vi "Dispose.vi"(8 "error in (no error)":errorcluster, 11 "STOMP in":refnum<class "STOMP.lvclass">) -> (0 "error out":errorcluster, 3 "STOMP out":refnum<class "STOMP.lvclass">)   [LabVIEW 2017, in "STOMP.lvclass"]
uses:
  STOMP.lvclass
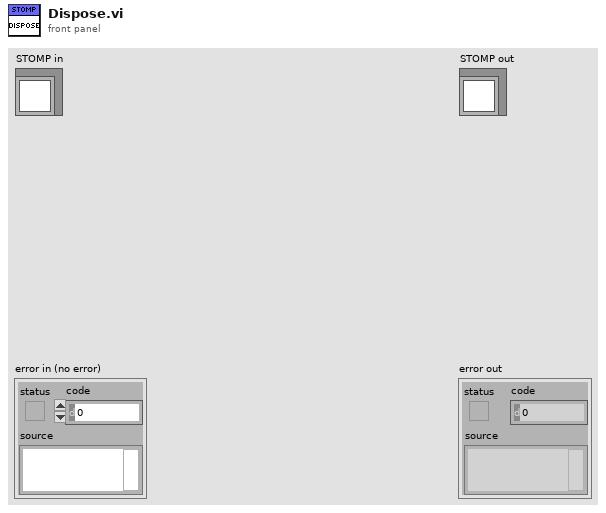
[diagram p1: front panel]
types:
  T1 = typedef "STOMP.lvclass/ObjectAttributes.ctl" = cluster{"address":string, "port":u16, "ConnectionRef":refnum<k5>, "messageQueue":refnum<queue>, "receiptQueue":refnum<queue>, "errorQueue":refnum<queue>, "sendQueue":refnum<queue>, "currentReceiptNumber":u64, "currentSubscriptionId":u64, "closeConnection":bool, "activeSubscriptions":T2[]}
  T2 = typedef "STOMP.lvclass/Type_ActiveSubscription.ctl" = cluster{"id":u64, "receipt":bool, "Destination":string, "ack":T3, "headers":T4[]}
  T3 = typedef "STOMP.lvclass/Type_AckHeader.ctl" = enum16{"auto", "client", "client-individual"}
  T4 = typedef "STOMP.lvclass/Type_FrameHeader.ctl" = cluster{"Header":string, "Value":string}
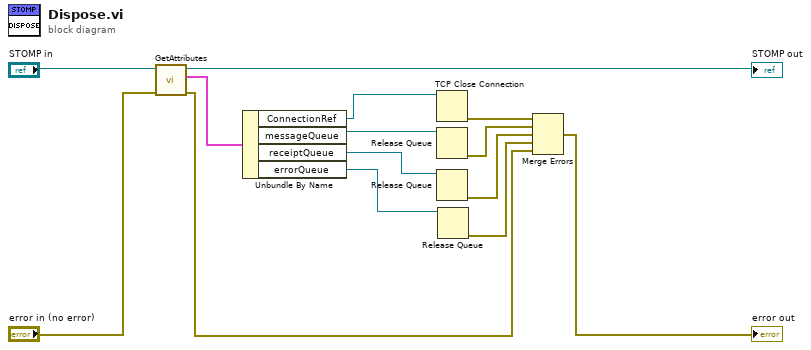
[diagram p0: block diagram]
diagram:
  n1 = call-dynamic "GetAttributes.vi"("error in (no error)"="error in (no error)", "STOMP in"="STOMP in") -> ("error out"=w1:errorcluster, "attributes"=w3:T1, "STOMP out"=→"STOMP out":refnum<class "STOMP.lvclass">)  [unwired: 7 in]
  n2 = Unbundle By Name(w3) -> ("ConnectionRef"=w11:refnum<k5>, "messageQueue"=w13:refnum<queue>, "receiptQueue"=w12:refnum<queue>, "errorQueue"=w14:refnum<queue>)
  n3 = TCP Close Connection(connection ID=w11) -> (error out=w10:errorcluster)  [unwired: 2 in, 1 out]
  n4 = Release Queue(queue=w13) -> (error out=w9:errorcluster)  [unwired: 2 in, 2 out]
  n5 = Release Queue(queue=w12) -> (error out=w8:errorcluster)  [unwired: 2 in, 2 out]
  n6 = Release Queue(queue=w14) -> (error out=w7:errorcluster)  [unwired: 2 in, 2 out]
  n7 = Merge Errors(w10, w9, w8, w7, w1) -> (→"error out":errorcluster)
